vi "Test-DotNet-Event.vi"() -> ()   [LabVIEW 2013, in "HardwareCharacterization.lvlib" / "HC-SM1000.lvclass"]
uses:
  HC-SM1000.lvclass
  DOTNET-settings.ctl
  Device-identification.ctl
  Fixed-data-type.ctl
  Status-information.ctl
  EC1000_DOTNET/handleConnectEvent.vi
  EC1000_DOTNET/getBroadcastData-status.vi
  C:/Users/vangeste/Desktop/2015-05-29 - SLM - MAIF/HC-HardwareCharacterization/Sources/SM1000/LECSession.dll
  LECSession.dll
panel:
  out "serverList iterator":i32
  out "Status information":T1
  out "Job count":i32
  out "Job name list":string
  out "Fixed data":string
  in  "File name wo extension":string="AdminConfig"
  in  "Fixed data type":T2=10 items=["Controller Configuration"=5, "Laser Configuration"=6, "Lens Configuration"=2, "Correction Table"=13, "User Configuration"=15, "Performance Adjustments"=16, "Admin Configuration"=10]
  in  "Device index":i32
  out "piServerCount":i32
  out "Device identifiers":T3[](array[typedef])
  in  "DOTNET settings":T4={"Target IP"="128.178.146.163", "Target broadcast port"=11000, "Target communication port"=12200, "clientID"=-1, "Broadcast IP"="224.168.100.2", "Servercount"=-1, "Device IDs"=[]}
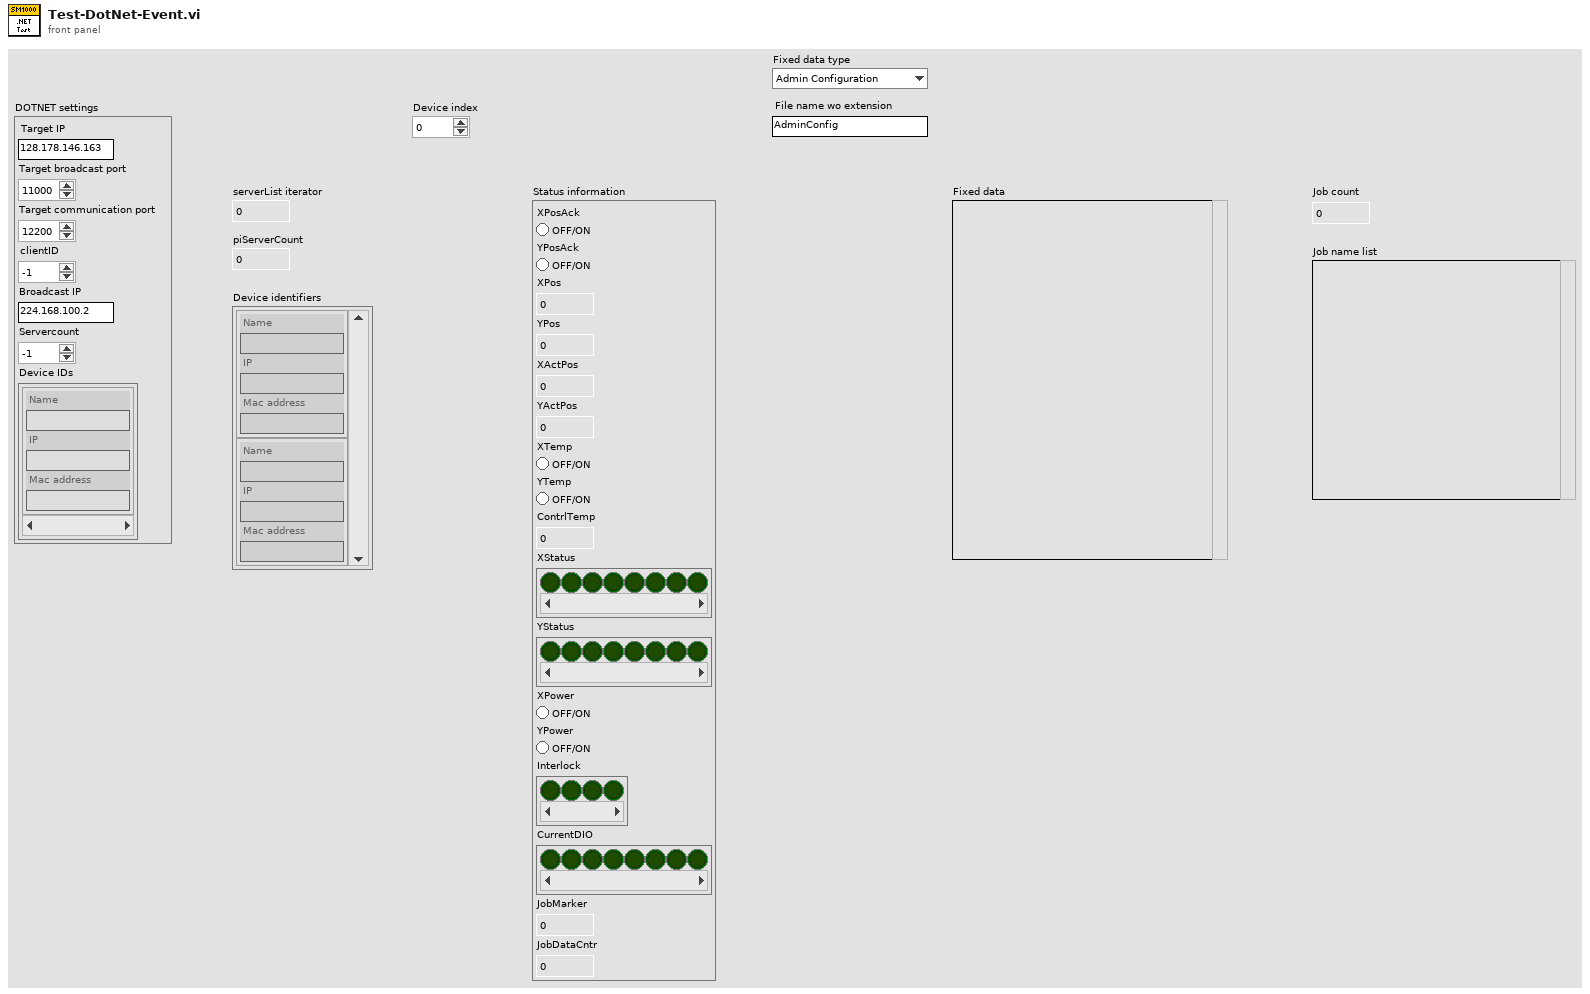
[diagram p1: front panel]
types:
  T1 = typedef "HardwareCharacterization.lvlib/HC-SM1000.lvclass/Status-information.ctl" = cluster{"XPosAck":bool, "YPosAck":bool, "XPos":i16, "YPos":i16, "XActPos":i16, "YActPos":i16, "XTemp":bool, "YTemp":bool, "ContrlTemp":i16, "XStatus":bool[], "YStatus":bool[], "XPower":bool, "YPower":bool, "Interlock":bool[], "CurrentDIO":bool[], "JobMarker":u16, "JobDataCntr":u32}
  T2 = typedef "HardwareCharacterization.lvlib/HC-SM1000.lvclass/Fixed-data-type.ctl" = i32
  T3 = typedef "HardwareCharacterization.lvlib/HC-SM1000.lvclass/Device-identification.ctl" = cluster{"Name":string, "IP":string, "Mac address":string}
  T4 = typedef "HardwareCharacterization.lvlib/HC-SM1000.lvclass/DOTNET-settings.ctl" = cluster{"Target IP":string, "Target broadcast port":i32, "Target communication port":i32, "clientID":i32, "Broadcast IP":string, "Servercount":i32, "Device IDs":T3[]}
  T5 = typedef "HardwareCharacterization.lvlib/HC-SM1000.lvclass/Object-reference.ctl" = refnum<data-value>
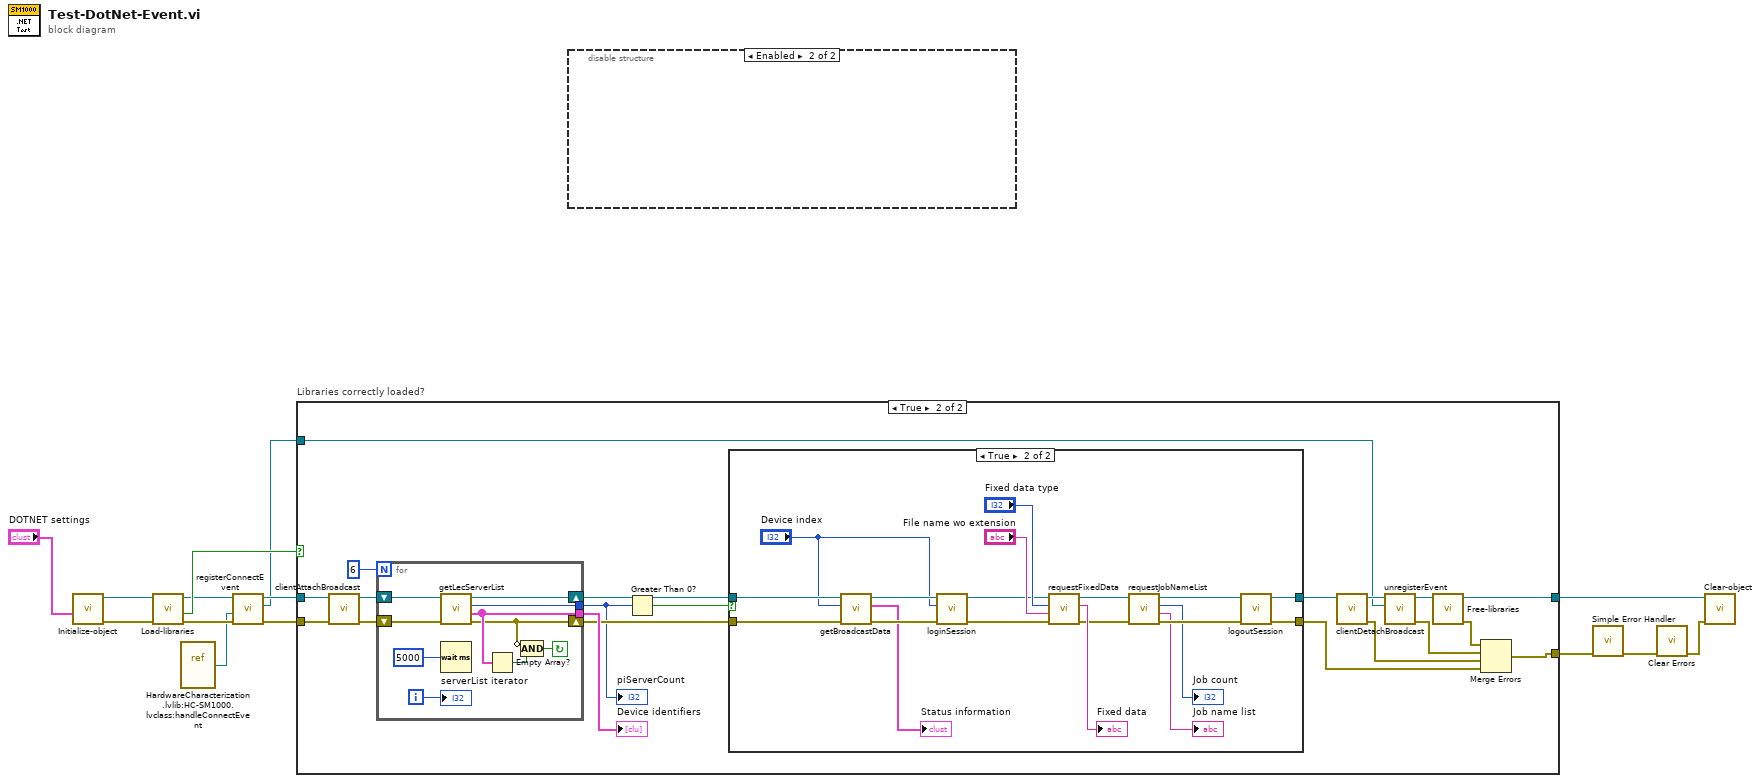
[diagram p0: block diagram]
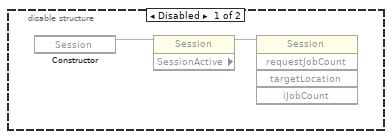
[diagram p2: hidden frame]
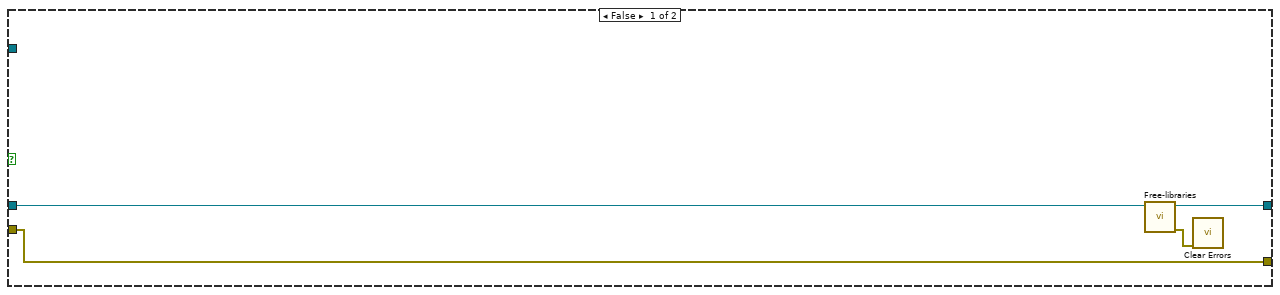
[diagram p3: hidden frame]
diagram:
  n1 = call "Initialize-object.vi"("DOTNET settings"="DOTNET settings") -> ("error out"=w12:errorcluster, "SM1000-control out"=w13:T5)  [unwired: 9 in]
  n2 = call "Load-libraries.vi"("error in (no error)"=w12, "SM1000-control in"=w13) -> ("error out"=w5:errorcluster, "Loaded?"=w11:bool, "SM1000-control out"=w6:T5)  [unwired: 7 in]
  n3 = vi-ref "HardwareCharacterization.lvlib:HC-SM1000.lvclass:handleConnectEvent.vi"() -> (w1:refnum<vi>)
  n4 = call "registerConnectEvent.vi"("error in (no error)"=w5, "Callback VI Ref"=w1, "SM1000-control in"=w6) -> ("error out"=w3:errorcluster, "Event Callback"=w2:refnum<k27>, "SM1000-control out"=w4:T5)  [unwired: 6 in]
  n5 = case "Libraries correctly loaded?" shown="True" w11 {
    tunnel: w4 -> [w17 w35]
    tunnel: w3 -> [w18 w34]
    tunnel: [w18 w37] -> w9
    tunnel: [w16 w36] -> w7
    tunnel: w2 -> [_ w19]
    frame False {
      n6 = call "Free-libraries.vi"("SM1000-control in"=w17) -> ("error out"=w15:errorcluster, "SM1000-control out"=w16:T5)  [unwired: 8 in, 1 out]
      n7 = call <vilib>:"Clear Errors.vi"("error in (no error)"=w15) -> ()  [unwired: 6 in, 1 out]
    }
    frame True {
      n8 = call "clientAttachBroadcast.vi"("error in (no error)"=w34, "SM1000-control in"=w35) -> ("error out"=w31:errorcluster, "SM1000-control out"=w32:T5)  [unwired: 7 in, 1 out]
      n9 = for {
        N: 6 -> [_]
        tunnel: [w64] -> w30
        tunnel: [w67] -> w24
        shift-right: [w66] -> w26
        shift-left: w32 -> [w69]
        shift-right: [w61] -> w25
        shift-left: w31 -> [w68]
        i -> [w63]
        stop <- w60 continue-if-true
        n10 = call "getLecServerList.vi"("error in (no error)"=w68, "SM1000-control in"=w69) -> ("error out"=w61:errorcluster, "Device identifiers"=w64:T3[], "piServerCount"=w67:i32, "SM1000-control out"=w66:T5)  [unwired: 6 in]
        n11 = Wait (ms)(milliseconds to wait=u32 5000) -> ()  [unwired: 1 out]
        n12 = Empty Array?(array=w64) -> (empty?=w62:bool)
        n13 = Compound Arithmetic op=AND(invert w61, w62) -> (w60:bool)
        "serverList iterator" <- w63
      }
      "Device identifiers" <- w30
      "piServerCount" <- w24
      n14 = Greater Than 0?(x=w24) -> (x > 0?=w23:bool)
      n15 = case shown="True" w23 {
        tunnel: [w39 w59] -> w28
        tunnel: [w40 w58] -> w27
        tunnel: w26 -> [w40 w46]
        tunnel: w25 -> [w39 w45]
        frame False {
        }
        frame True {
          n16 = call-poly "getBroadcastData.vi"("error in (no error)"=w45, "Device index"="Device index", "SM1000-control in"=w46) -> ("error out"=w43:errorcluster, "Status information"=→"Status information":T1, "SM1000-control out"=w44:T5)  [unwired: 6 in]
          n17 = call "loginSession.vi"("error in (no error)"=w43, "Device index"="Device index", "SM1000-control in"=w44) -> ("error out"=w54:errorcluster, "SM1000-control out"=w55:T5)  [unwired: 7 in]
          n18 = call "requestFixedData.vi"("error in (no error)"=w54, "File name wo extension"="File name wo extension", "Fixed data type"="Fixed data type", "SM1000-control in"=w55) -> ("error out"=w51:errorcluster, "File contents"=→"Fixed data":string, "SM1000-control out"=w52:T5)  [unwired: 5 in]
          n19 = call "requestJobNameList.vi"("error in (no error)"=w51, "SM1000-control in"=w52) -> ("error out"=w49:errorcluster, "Job name list"=→"Job name list":string, "Job count"=→"Job count":i32, "SM1000-control out"=w50:T5)  [unwired: 6 in]
          n20 = call "logoutSession.vi"("error in (no error)"=w49, "SM1000-control in"=w50) -> ("error out"=w59:errorcluster, "SM1000-control out"=w58:T5)  [unwired: 8 in]
        }
      }
      n21 = call "clientDetachBroadcast.vi"("SM1000-control in"=w27) -> ("error out"=w33:errorcluster, "SM1000-control out"=w22:T5)  [unwired: 9 in]
      n22 = call "unregisterEvent.vi"("Event Callback in"=w19, "SM1000-control in"=w22) -> ("error out"=w20:errorcluster, "SM1000-control out"=w21:T5)  [unwired: 8 in]
      n23 = call "Free-libraries.vi"("SM1000-control in"=w21) -> ("error out"=w38:errorcluster, "SM1000-control out"=w36:T5)  [unwired: 8 in, 1 out]
      n24 = Merge Errors(w38, w20, w33, w28) -> (w37:errorcluster)
    }
  }
  n25 = disable-structure shown="Enabled" {
    frame Disabled {
      n26 = constructor class="Session"() -> (reference out=w71:refnum<k24>)  [unwired: 3 in, 2 out]
      n27 = property class="Session" props=["SessionActive"](reference=w71) -> (reference out=w70:refnum<k24>)  [unwired: 1 in, 2 out]
      n28 = invoke class="Session" method="requestJobCount"(reference=w70) -> ()  [unwired: 4 in, 5 out]
    }
    frame Enabled {
    }
  }
  n29 = call <vilib>:"Simple Error Handler.vi"("error in (no error)"=w9) -> ("error out"=w10:errorcluster)  [unwired: 4 in, 4 out]
  n30 = call <vilib>:"Clear Errors.vi"("error in (no error)"=w10) -> ("error out"=w8:errorcluster)  [unwired: 6 in]
  n31 = call "Clear-object.vi"("error in (no error)"=w8, "SM1000-control"=w7) -> ()  [unwired: 8 in, 2 out]
